vi "Login Screens.vi"() -> ()   [LabVIEW 2021]
panel:
  in  "PASSWORD":string
  in  "ROLES":string(combo)
  in  "USERNAME":string
  in  "Close Button":bool
  in  "OK Button":bool
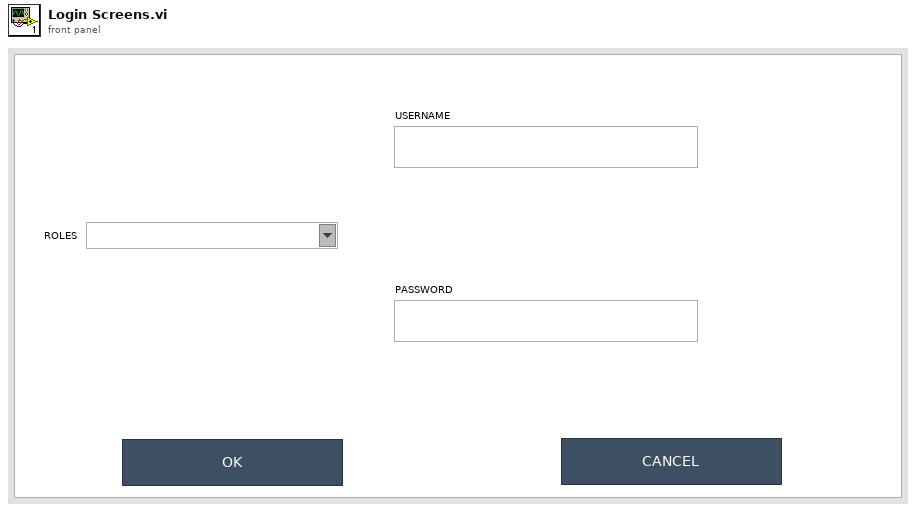
[diagram p1: front panel]
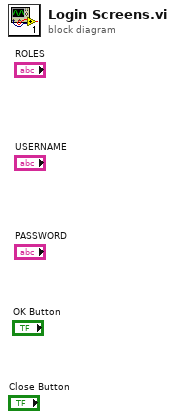
[diagram p0: block diagram]
diagram:
